vi "Auto Resource.vi"(8 "error in (no error)":errorcluster, 11 "DeployTarget in":refnum<class "Platform.lvclass">) -> (0 "error out":errorcluster, 2 "Auto Resource":bool, 3 "DeployTarget out":refnum<class "Platform.lvclass">)   [LabVIEW 2020, in "PicoG-Core.lvlib" / "Platform.lvclass"]
uses:
  Platform.lvclass
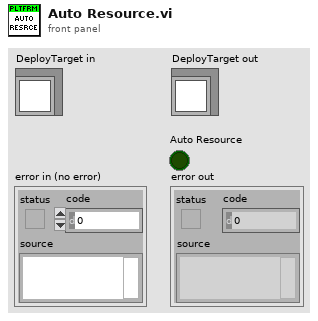
[diagram p1: front panel]
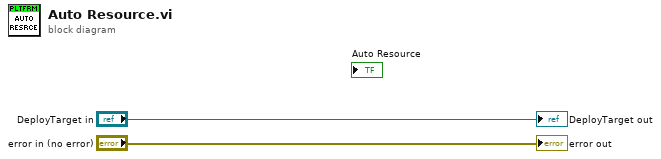
[diagram p0: block diagram]
diagram:
  "error out" <- "error in (no error)"
  "DeployTarget out" <- "DeployTarget in"
